vi "Brk_Pt_Trig_NoBuffer.vi"(0 "Board ID":T3=1 min=1 max=32 step=1, 1 "Axis":T1=1 items=["Axis 1"=1, "Axis 2"=2, "Axis 3"=3, "Axis 4"=4, "Axis 5"=5, "Axis 6"=6, "Axis 7"=7, "Axis 8"=8], 2 "Reverse ?":bool, 5 "Number of steps":i32=10, 11 "error in (no error)":errorcluster, 12 "Total steps":i32) -> (4 "Start Position":i32, 6 "End Position":i32, 10 "Motion error":bool)   [LabVIEW 2022 SP3]
doc: "EXAMPLE: DO_WHILE Loop (Onboard Programming Template)\n\nSUMMARY:\nThis FlexMotion example demonstrates the implementation of a DO_WHILE loop data structure in an onboard program. The C equivalent of the data structure implemented here is:\n\ndo {\n// code to be repeated\nloopVar = loopVar - increment;\n} while (loopVar != 0);\n\nTHEORY OF OPERATION:\nThe flow of the DO_WHILE loop data structure goes as follows:\n(1) Program storage is begun.\n(2) The DO_WHILE loop is set up. (Loop Variable and Increment are each defined and initialized.)\n(3) A code delimiter is set using label #1.\n(4) Code to be executed each time through loop is run (in the template program, the loop variable is decremented).\n(5) The loop variable or other test condition is checked.\n(6) If the test condition is true, then we jump back to label #1. Otherwise, the condition is false so the loop terminates.\n(7) Program storage is ended.\n\nDEVELOPMENT DETAILS:\nApplication Software: LabVIEW 5.0.x\nHardware: FlexMotion controller\nDriver Software: FlexMotion Software 4.0\n\nREQUIRED HARDWARE:\n(controller only)\n\nINSTRUCTIONS:\n(0) Initialize the FlexMotion controller before running this VI. \n(1) Add the FlexMotion functions you want to execute into the block diagram where noted.\n(2) Run the VI to store the program. (The program will not be executed at this time.)\n(3) You can then run the program you have stored by calling the run_prog.flx function with the appropriate program number.\n\nADDITIONAL NOTES:\n(a) You should read the following items before writing FlexMotion onboard programs:\n(1) The Onboard Programs section of the FlexMotion Hardware User Manual (page 4-9 in the November 1998 edition).\n(2) The section about onboard variables in your FlexMotion Software Reference Manual (pages 4-11 and 4-12 in the November 1998 edition)\n(3) You will find the chapter of the FlexMotion Software Reference Manual concerning the Onboard Programming functions to be an invaluable reference resource (Chapter 12 of the November 1998 edition) along with the online help for the VI functions.\n(b) This template repeats the DO_WHILE loop as long as an expression with a variable evaluates to be true. However, you may evaluate other conditions such as move complete status instead.\n\n*NOTE: This example is not supported on the 7334 controller."
uses:
  -MotionRoutines/MotionGlobals.vi
  <vilib>/Motion/FlexMotion/FunctionsVIs/StartStopMotion.llb/Start Motion (8 axes).flx
  <vilib>/Motion/FlexMotion/FunctionsVIs/OnboardProgramming.llb/Jump to Label on Condition (8 axes).flx
  <vilib>/Motion/FlexMotion/FunctionsVIs/Trajectory.llb/Load Acceleration/Deceleration.flx
  <vilib>/Motion/FlexMotion/FunctionsVIs/MotionIO.llb/Set Breakpoint Output MOMO (8 axes).flx
  <vilib>/Motion/FlexMotion/CustomControls/CustomControls.llb/Mask (8 axes).flx
  <vilib>/Motion/FlexMotion/CustomControls/CustomControls.llb/MustOn (8 axes).flx
  <vilib>/Motion/FlexMotion/CustomControls/CustomControls.llb/Program.flx
  <vilib>/Motion/FlexMotion/CustomControls/CustomControls.llb/Axis To Read.flx
panel:
  out "Store Loop":i32
  out "Done loop":i32
  out "Motion stop loop":i32
  in  "Program (1)":T2=1 format="%.0x"
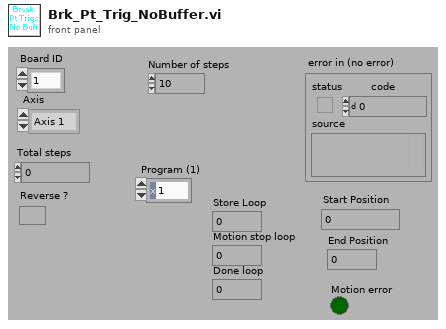
[diagram p1: front panel]
types:
  T1 = typedef "Axis To Read.flx" = u16
  T2 = typedef "Program.flx" = u8
  T3 = typedef "Board Id" = u8
  T4 = enum16{"No Change", "Reset on Breakpoint", "Set on Breakpoint", "Toggle on Breakpoint", "Create Pulse on Breakpoint"}
  T5 = typedef "Mask (8 axes).flx" = cluster{"1":bool, "2":bool, "3":bool, "4":bool, "5":bool, "6":bool, "7":bool, "8":bool}
  T6 = typedef "MustOn (8 axes).flx" = cluster{"0":bool, "1":bool, "2":bool, "3":bool, "4":bool, "5":bool, "6":bool, "7":bool, "8":bool}
  T7 = enum16{"Less Than", "Equal", "Less Than Or Equal", "Greater Than", "Not Equal", "Greater Than Or Equal", "True", "Home Found", "Index Found", "High Speed Capture", "Position Breakpoint", "Reserved", "Velocity Threshold", "Move Complete", "Profile Complete", "Blend Complete", "Motor Off", "Home Input Active", "Limit Input Active", "Software Limit Active", "Program Complete", "IO Port Match"}
  T8 = typedef "Var" = u8
  T9 = typedef "Bd Id Out" = u8
  T10 = typedef "Resource Out (Enum).flx" = u16
  T11 = cluster{"Reserved":bool, "Axis #1 Move Complete":bool, "Axis #2 Move Complete":bool, "Axis #3 Move Complete":bool, "Axis #4 Move Complete":bool, "Axis #5 Move Complete":bool, "Axis #6 Move Complete":bool, "Axis #7 Move Complete":bool, "Axis #8 Move Complete":bool, "Axis #9 MoveComplete":bool, "Axis #10 Move Complete":bool, "Axis #11 Move Complete":bool, "Axis #12 Move Complete":bool, "Status #13":bool, "Status #14":bool, "Status #15":bool}
  T12 = cluster{"Run/Stop":bool, "Profile Complete":bool, "Motor Off ":bool, "Following Error":bool, "Limit Switch":bool, "Home Switch":bool, "SW Limit Switch":bool, "Watchdog":bool, "Velocity Threshold":bool, "Position Brkpt":bool, "Home Found":bool, "Index Found":bool, "High Speed Capture":bool, "Reverse Direction":bool, "Blend Complete":bool, "Move Complete":bool}
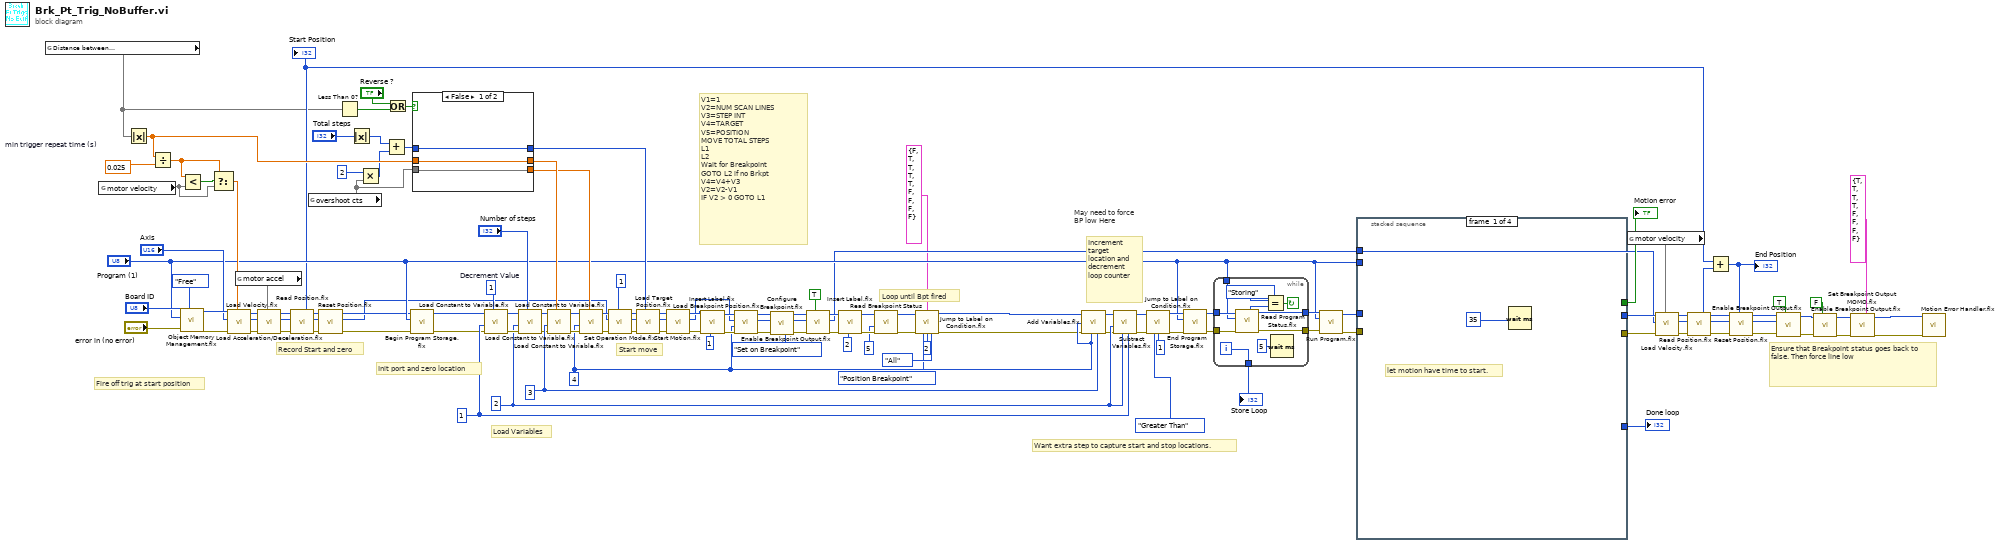
[diagram p0: block diagram]
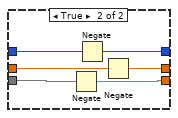
[diagram p2: hidden frame]
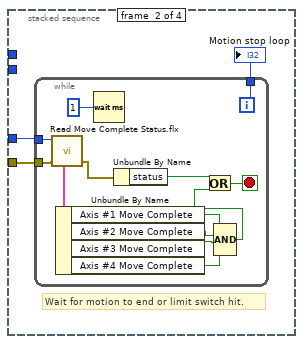
[diagram p3: hidden frame]
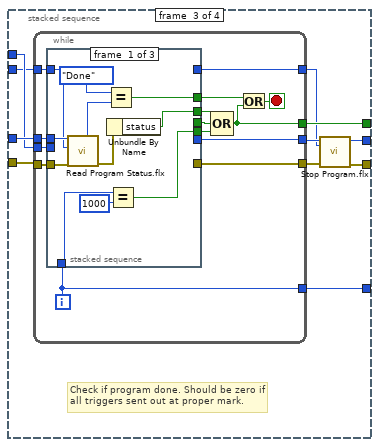
[diagram p4: hidden frame]
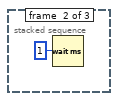
[diagram p5: hidden frame]
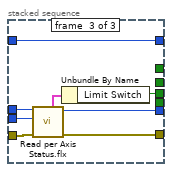
[diagram p6: hidden frame]
diagram:
  w83 = 0.025  # min trigger repeat time (s)
  w57 = T8 4 ("Step Int Variable")
  w114 = T8 3 ("Step Int Variable")
  w121 = T8 2 ("Loop Variable")
  w122 = T8 1 ("Decrement Variable")
  w123 = 1  # Decrement Value
  # "Ensure that Breakpoint status goes back to false. Then force line low"
  # "Fire off trig at start position"
  # "V1=1\nV2=NUM SCAN LINES\nV3=STEP INT\nV4=TARGET\nV5=POSITION\nMOVE TOTAL STEPS\nL1\nL2\nWait for Breakpoint\nGOTO L2 if no Brkpt\nV4=V4+V3\nV2=V2-V1\nIF V2 > 0 GOTO L1"
  # "Record Start and zero"
  # "Init port and zero location"
  # "Load Variables"
  # "Start move"
  # "Increment target location and decrement loop counter"
  # "Loop until Bpt fired"
  # "Want extra step to capture start and stop locations."
  # "May need to force BP low Here"
  n1 = global read "MotionGlobals.vi" "Distance between\nscan lines (mm)"() -> (w1)
  n2 = global read "MotionGlobals.vi" "motor velocity"() -> (w72)
  n3 = Absolute Value(x=w1) -> (abs(x)=w75:dbl)
  n4 = Divide(x=w75, y=w83) -> (x/y=w81:dbl)
  n5 = call <vilib>:"Object Memory Management.flx"("Operation"=enum16{"Save", "Delete", "Free"}."Free" ("Operation (Free)"), "error in (no error)"="error in (no error)", "Object (1)"="Program (1)", "Board ID"="Board ID") -> ("error out"=w62:errorcluster, "Bd ID Out"=w61:T9)  [unwired: 4 out]
  n6 = Less?(x=w81, y=w72) -> (x < y?=w82:bool)
  n7 = Select(t=w81, s=w82, f=w72) -> (s? t:f=w79:dbl)
  n8 = call <vilib>:"Load Velocity.flx"("Velocity (10000)"=w79, "error in (no error)"=w62, "Axis or Vector Space"="Axis", "Board ID"=w61) -> ("error out"=w69:errorcluster, "Resource Output"=w66:T10, "Bd ID Out"=w68:T9)  [unwired: 3 out]
  n9 = global read "MotionGlobals.vi" "motor accel"() -> (w67)
  n10 = call "Load Acceleration/Deceleration.flx"("Acceleration (100000)"=w67, "error in (no error)"=w69, "Axis or Vector Space"=w66, "Board ID"=w68) -> ("error out"=w70:errorcluster, "Resource Output"=w63:T10, "Bd ID Out"=w71:T9)  [unwired: 1 in, 2 out]
  n11 = call <vilib>:"Read Position.flx"("error in (no error)"=w70, "Axis"=w63, "Board ID"=w71) -> ("error out"=w102:errorcluster, "Resource Output"=w101:T10, "Bd ID Out"=w103:T9, "Position"=w32:i32)  [unwired: 3 out]
  "Start Position" <- w32
  n12 = global read "MotionGlobals.vi" "overshoot cts"() -> (w2)
  n13 = call <vilib>:"Reset Position.flx"("error in (no error)"=w102, "Axis"=w101, "Board ID"=w103) -> ("error out"=w7:errorcluster, "Resource Output"=w5:T10, "Bd ID Out"=w6:T9)  [unwired: 2 in, 2 out]
  n14 = Less Than 0?(x=w1) -> (x < 0?=w78:bool)
  n15 = Absolute Value(x="Total steps") -> (abs(x)=w52:i32)
  n16 = Multiply(x=2, y=w2) -> (x*y=w4:i32)
  n17 = Add(x=w52, y=w4) -> (x+y=w53:i32)
  n18 = Or(x="Reverse ?", y=w78) -> (x .or. y?=w76:bool)
  n19 = call <vilib>:"Begin Program Storage.flx"("error in (no error)"=w7, "Program (1)"="Program (1)", "Board ID"=w6) -> ("error out"=w99:errorcluster, "Bd ID Out"=w100:T9)  [unwired: 4 out]
  n20 = case shown="False" w76 {
    tunnel: w53 -> [w135 w141]
    tunnel: [w135 w140] -> w87
    tunnel: [w134 w138] -> w60
    tunnel: w75 -> [w134 w139]
    tunnel: w2 -> [w133 w137]
    tunnel: [w133 w136] -> w51
    frame False {
    }
    frame True {
      n21 = Negate(x=w137) -> (-x=w136:dbl)
      n22 = Negate(x=w141) -> (-x=w140:i32)
      n23 = Negate(x=w139) -> (-x=w138:dbl)
    }
  }
  n24 = call <vilib>:"Load Constant to Variable.flx"("Value (0)"=w123, "error in (no error)"=w99, "Var"=w122, "Board ID"=w100) -> ("error out"=w126:errorcluster, "Bd ID Out"=w128:T9)  [unwired: 4 out]
  n25 = call <vilib>:"Load Constant to Variable.flx"("Value (0)"="Number of steps", "error in (no error)"=w126, "Var"=w121, "Board ID"=w128) -> ("error out"=w112:errorcluster, "Bd ID Out"=w113:T9)  [unwired: 4 out]
  n26 = call <vilib>:"Load Constant to Variable.flx"("Value (0)"=w60, "error in (no error)"=w112, "Var"=w114, "Board ID"=w113) -> ("error out"=w115:errorcluster, "Bd ID Out"=w116:T9)  [unwired: 4 out]
  n27 = call <vilib>:"Load Constant to Variable.flx"("Value (0)"=w51, "error in (no error)"=w115, "Var"=w57, "Board ID"=w116) -> ("error out"=w108:errorcluster, "Bd ID Out"=w109:T9)  [unwired: 4 out]
  n28 = call <vilib>:"Set Operation Mode.flx"("Position Mode (Absolute)"=1, "error in (no error)"=w108, "Axis or Vector Space"=w5, "Board ID"=w109) -> ("error out"=w106:errorcluster, "Resource Output"=w98:T10, "Bd ID Out"=w107:T9)  [unwired: 2 out]
  n29 = call <vilib>:"Load Target Position.flx"("Target Position (0)"=w87, "error in (no error)"=w106, "Axis"=w98, "Board ID"=w107) -> ("error out"=w110:errorcluster, "Resource Output"=w111:T10, "Bd ID Out"=w104:T9)  [unwired: 3 out]
  n30 = call-poly <vilib>:"Start Motion.flx"("error in (no error)"=w110, "Axis or Vector Space"=w111, "Board ID"=w104) -> ("error out"=w94:errorcluster, "Resource Output"=w48:T10, "Bd ID Out"=w95:T9)  [unwired: 1 in, 2 out]
  n31 = call <vilib>:"Insert Label.flx"("Label Number (1)"=u16 1 ("Label"), "error in (no error)"=w94, "Board ID"=w95) -> ("error out"=w58:errorcluster, "Bd ID Out"=w59:T9)  [unwired: 4 out]
  n32 = call <vilib>:"Load Breakpoint Position.flx"("error in (no error)"=w58, "Inp Vect"=w57, "Axis or Encoder"=w48, "Board ID"=w59) -> ("error out"=w24:errorcluster, "Resource Output"=w20:T10, "Bd ID Out"=w19:T9)  [unwired: 1 in, 2 out]
  n33 = call <vilib>:"Configure Breakpoint.flx"("Action (No Change)"=T4."Set on Breakpoint", "error in (no error)"=w24, "Axis or Encoder"=w20, "Board ID"=w19) -> ("error out"=w23:errorcluster, "Resource Output"=w21:T10, "Bd ID Out"=w22:T9)  [unwired: 2 in, 3 out]
  n34 = call <vilib>:"Enable Breakpoint Output.flx"("Enable Breakpoint"=TRUE, "error in (no error)"=w23, "Axis or Encoder"=w21, "Board ID"=w22) -> ("error out"=w55:errorcluster, "Resource Output"=w17:T10, "Bd ID Out"=w56:T9)  [unwired: 3 out]
  n35 = call <vilib>:"Insert Label.flx"("Label Number (1)"=u16 2 ("Label"), "error in (no error)"=w55, "Board ID"=w56) -> ("error out"=w49:errorcluster, "Bd ID Out"=w50:T9)  [unwired: 4 out]
  n36 = call <vilib>:"Read Breakpoint Status.vi"("error in (no error)"=w49, "Ret Vect"=5, "Board ID"=w50) -> ("error out"=w43:errorcluster, "Bd ID Out"=w44:T9)  [unwired: 2 in, 3 out]
  n37 = call-poly <vilib>:"Jump to Label on Condition.flx"("Board ID"=w44, "Must Off (False)"=T6 {"0"=FALSE, "1"=TRUE, "2"=TRUE, "3"=TRUE, "4"=TRUE, "5"=FALSE, "6"=FALSE, "7"=FALSE, "8"=FALSE}, "error in (no error)"=w43, "Condition Code (True)"=T7."Position Breakpoint", "Jump to Label (1)"=u16 2, "Match Type (All)"=enum16{"All", "Any"}."All") -> ("Bd ID Out"=w9:T9, "error out"=w8:errorcluster)  [unwired: 2 in, 6 out]
  n38 = call <vilib>:"Add Variables.flx"("Var 2"=w114, "Var 1"=w57, "error in (no error)"=w8, "Ret Vect"=w57, "Board ID"=w9) -> ("error out"=w118:errorcluster, "Bd ID Out"=w117:T9)  [unwired: 3 out]
  n39 = call <vilib>:"Subtract Variables.flx"("Var 2"=w122, "Var 1"=w121, "error in (no error)"=w118, "Ret Vect"=w121, "Board ID"=w117) -> ("error out"=w124:errorcluster, "Bd ID Out"=w127:T9)  [unwired: 3 out]
  n40 = call-poly <vilib>:"Jump to Label on Condition.flx"("Board ID"=w127, "error in (no error)"=w124, "Condition Code (True)"=T7."Greater Than", "Jump to Label (1)"=u16 1) -> ("Bd ID Out"=w131:T9, "error out"=w125:errorcluster)  [unwired: 4 in, 6 out]
  n41 = call <vilib>:"End Program Storage.flx"("error in (no error)"=w125, "Program (1)"="Program (1)", "Board ID"=w131) -> ("error out"=w91:errorcluster, "Bd ID Out"=w92:T9)  [unwired: 4 out]
  n42 = while {
    tunnel: w92 -> [w151]
    tunnel: w91 -> [w150]
    tunnel: [w149] -> w90
    tunnel: [w148] -> w89
    tunnel: "Program (1)" -> [w147]
    tunnel: [w143] -> w88
    i -> [w143]
    stop <- w144 continue-if-true
    n43 = call <vilib>:"Read Program Status.flx"("error in (no error)"=w150, "Program (1)"=w147, "Board Id"=w151) -> ("error out"=w148:errorcluster, "Bd Id Out"=w149:T9, "Program Status"=w145:enum16{"Done", "Playing", "Paused", "Storing"})  [unwired: 4 out]
    n44 = Equal?(x=enum16{"Done", "Playing", "Paused", "Storing"}."Storing" ("Program Status"), y=w145) -> (x = y?=w144:bool)
    n45 = Wait (ms)(milliseconds to wait=5) -> ()  [unwired: 1 out]
  }
  "Store Loop" <- w88
  n46 = call <vilib>:"Run Program.flx"("error in (no error)"=w89, "Program (1)"="Program (1)", "Board ID"=w90) -> ("error out"=w96:errorcluster, "Bd ID Out"=w97:T9)  [unwired: 4 out]
  n47 = stacked-sequence {
    tunnel: w97 -> [_ w155 w179 _]
    tunnel: w96 -> [_ w153 w178 _]
    tunnel: [_ _ w176 _] -> w86
    tunnel: [_ _ w175 _] -> w85
    tunnel: w17 -> [_ _ w174 _]
    tunnel: "Program (1)" -> [_ _ w173 _]
    tunnel: [_ _ w171 _] -> w74
    tunnel: [_ _ w170 _] -> w73
    frame #0 {
      # "let motion have time to start."
      n48 = Wait (ms)(milliseconds to wait=35) -> ()  [unwired: 1 out]
    }
    frame #1 {
      # "Wait for motion to end or limit switch hit."
      n49 = while {
        tunnel: w155 -> [w168]
        tunnel: [w157] -> w154
        tunnel: w153 -> [w156]
        i -> [w157]
        stop <- w159 stop-if-true
        n50 = call <vilib>:"Read Move Complete Status.flx"("error in (no error)"=w156, "Board ID"=w168) -> ("error out"=w167:errorcluster, "Move Complete Status"=w166:T11)  [unwired: 1 in, 4 out]
        n51 = Unbundle By Name(w166) -> ("Axis #1 Move Complete"=w162:bool, "Axis #2 Move Complete"=w165:bool, "Axis #3 Move Complete"=w164:bool, "Axis #4 Move Complete"=w163:bool)
        n52 = Wait (ms)(milliseconds to wait=1) -> ()  [unwired: 1 out]
        n53 = Unbundle By Name(w167) -> ("status"=w161:bool)
        n54 = Compound Arithmetic op=AND(w162, w165, w164, w163) -> (w160:bool)
        n55 = Or(x=w161, y=w160) -> (x .or. y?=w159:bool)
      }
      "Motion stop loop" <- w154
    }
    frame #2 {
      # "Check if program done. Should be zero if all triggers sent out at proper mark."
      n56 = while {
        tunnel: w178 -> [w190]
        tunnel: [w193] -> w172
        tunnel: [w192] -> w177
        tunnel: w179 -> [w191]
        tunnel: [w185] -> w176
        tunnel: [w183] -> w175
        tunnel: w174 -> [w182]
        tunnel: w173 -> [w181]
        tunnel: [w180] -> w169
        i -> [w183]
        stop <- w186 stop-if-true
        n57 = stacked-sequence {
          tunnel: [_ _ w208] -> w193
          tunnel: [_ _ w209] -> w192
          tunnel: w191 -> [w196 _ w212]
          tunnel: w190 -> [w195 _ w211]
          tunnel: [w201 _ _] -> w189
          tunnel: [_ _ w210] -> w188
          tunnel: [w200 _ _] -> w187
          tunnel: w183 -> [w199 _ _]
          tunnel: [w197 _ _] -> w184
          tunnel: w182 -> [_ _ w207]
          tunnel: w181 -> [w194 _ w206]
          tunnel: [_ _ w206] -> w180
          frame #0 {
            n58 = call <vilib>:"Read Program Status.flx"("error in (no error)"=w195, "Program (1)"=w194, "Board Id"=w196) -> ("error out"=w202:errorcluster, "Program Status"=w203:enum16{"Done", "Playing", "Paused", "Storing"})  [unwired: 5 out]
            n59 = Equal?(x=enum16{"Done", "Playing", "Paused", "Storing"}."Done" ("Program Status"), y=w203) -> (x = y?=w200:bool)
            n60 = Unbundle By Name(w202) -> ("status"=w201:bool)
            n61 = Equal?(x=w199, y=1000) -> (x = y?=w197:bool)
          }
          frame #1 {
            n62 = Wait (ms)(milliseconds to wait=1) -> ()  [unwired: 1 out]
          }
          frame #2 {
            n63 = call <vilib>:"Read per Axis Status.flx"("error in (no error)"=w211, "Axis"=w207, "Board ID"=w212) -> ("error out"=w209:errorcluster, "Bd ID Out"=w208:T9, "Per Axis H/W Status"=w213:T12)  [unwired: 4 out]
            n64 = Unbundle By Name(w213) -> ("Limit Switch"=w210:bool)
          }
        }
        n65 = Compound Arithmetic op=OR(w189, w188, w184) -> (w185:bool)
        n66 = Or(x=w187, y=w185) -> (x .or. y?=w186:bool)
      }
      n67 = call <vilib>:"Stop Program.flx"("error in (no error)"=w177, "Program (1)"=w169, "Board ID"=w172) -> ("error out"=w170:errorcluster, "Bd ID Out"=w171:T9)  [unwired: 4 out]
    }
    frame #3 {
      # "Add extra triggers in case of a missed trigger or two."
    }
  }
  "Motion error" <- w86
  "Done loop" <- w85
  n68 = global read "MotionGlobals.vi" "motor velocity"() -> (w80)
  n69 = call <vilib>:"Load Velocity.flx"("Velocity (10000)"=w80, "error in (no error)"=w73, "Axis or Vector Space"=w17, "Board ID"=w74) -> ("error out"=w37:errorcluster, "Resource Output"=w34:T10, "Bd ID Out"=w38:T9)  [unwired: 3 out]
  n70 = call <vilib>:"Read Position.flx"("error in (no error)"=w37, "Axis"=w34, "Board ID"=w38) -> ("error out"=w39:errorcluster, "Resource Output"=w35:T10, "Bd ID Out"=w36:T9, "Position"=w33:i32)  [unwired: 3 out]
  n71 = Add(x=w32, y=w33) -> (x+y=w31:i32)
  "End Position" <- w31
  n72 = call <vilib>:"Reset Position.flx"("Primary Reset Position (0)"=w31, "error in (no error)"=w39, "Axis"=w35, "Board ID"=w36) -> ("error out"=w29:errorcluster, "Resource Output"=w26:T10, "Bd ID Out"=w30:T9)  [unwired: 1 in, 2 out]
  n73 = call <vilib>:"Enable Breakpoint Output.flx"("Enable Breakpoint"=TRUE, "error in (no error)"=w29, "Axis or Encoder"=w26, "Board ID"=w30) -> ("error out"=w14:errorcluster, "Bd ID Out"=w15:T9)  [unwired: 4 out]
  n74 = call <vilib>:"Enable Breakpoint Output.flx"("Enable Breakpoint"=FALSE, "error in (no error)"=w14, "Board ID"=w15) -> ("error out"=w12:errorcluster, "Bd ID Out"=w13:T9)  [unwired: 1 in, 4 out]
  n75 = call-poly <vilib>:"Set Breakpoint Output MOMO.flx"("Must Off (False)"=T5 {"1"=TRUE, "2"=TRUE, "3"=TRUE, "4"=TRUE, "5"=FALSE, "6"=FALSE, "7"=FALSE, "8"=FALSE}, "error in (no error)"=w12, "Board ID"=w13) -> ("error out"=w27:errorcluster, "Bd ID Out"=w28:T9)  [unwired: 3 in, 2 out]
  n76 = call <vilib>:"Motion Error Handler.flx"("Board ID"=w28, "error in (no error)"=w27) -> ()  [unwired: 3 in, 11 out]
